vi "float_To_String.vi"() -> ()   [LabVIEW 2020]
panel:
  out "String 2":string
  out "String":string
  in  "Numeric":dbl
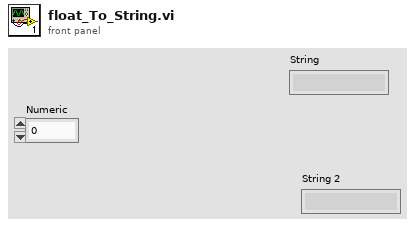
[diagram p1: front panel]
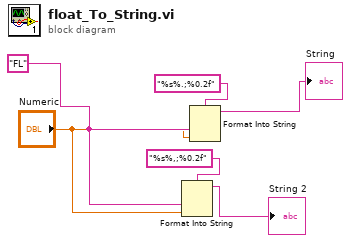
[diagram p0: block diagram]
diagram:
  w2 = "FL" ("Command")
  n1 = Format Into String(format string="%s%,;%0.2f" ("Format String"), w2, "Numeric") -> (resulting string=→"String 2":string)  [unwired: 2 in, 1 out]
  n2 = Format Into String(format string="%s%.;%0.2f" ("Format String"), w2, "Numeric") -> (resulting string=→"String":string)  [unwired: 2 in, 1 out]
